vi "SVA 4MV6 P001 CCE histograma colores.vi"(11 "Image":T1) -> (1 "HGB":u8[](array[numeric]), 2 "HGG":u8[](array[numeric]), 3 "HGR":u8[](array[numeric]))   [LabVIEW 2020]
uses:
  <vilib>/vision/Image Controls.llb/IMAQ Image.ctl
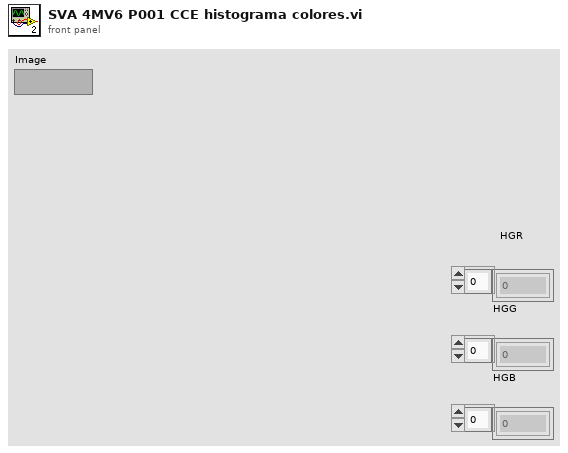
[diagram p1: front panel]
types:
  T1 = typedef "IMAQ Image.ctl" = refnum<image>
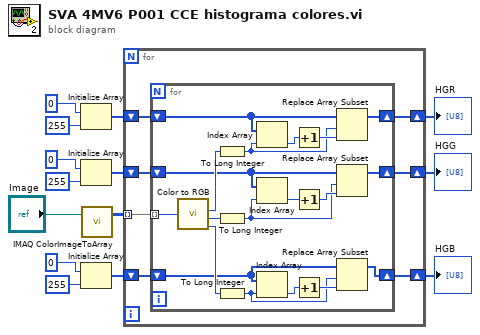
[diagram p0: block diagram]
diagram:
  n1 = Initialize Array(u8 0 ("element"), 255 ("dimension size")) -> (w12:u8[])
  n2 = Initialize Array(u8 0 ("element"), 255 ("dimension size")) -> (w6:u8[])
  n3 = Initialize Array(u8 0 ("element"), 255 ("dimension size")) -> (w5:u8[])
  n4 = call "IMAQ ColorImageToArray"("Image"="Image") -> ("Image Pixels (U32)"=w11:u32[][])  [unwired: 3 in, 2 out]
  n5 = for {
    shift-right: [w20] -> w4
    shift-left: w12 -> [w21]
    tunnel: w11 -> [w19] mode=indexing
    shift-right: [w17] -> w3
    shift-left: w6 -> [w18]
    shift-right: [w15] -> w2
    shift-left: w5 -> [w16]
    n6 = for {
      shift-right: [w37] -> w20
      shift-left: w21 -> [w38]
      tunnel: w19 -> [w36] mode=indexing
      shift-right: [w28] -> w17
      shift-left: w18 -> [w30]
      shift-right: [w22] -> w15
      shift-left: w16 -> [w23]
      n7 = call <vilib>:"Color to RGB.vi"("Color"=w36) -> ("R"=w35:u8, "G"=w29:u8, "B"=w24:u8)  [unwired: 1 out]
      n8 = To Long Integer(number=w35) -> (32bit integer=w34:i32)
      n9 = To Long Integer(number=w29) -> (32bit integer=w31:i32)
      n10 = To Long Integer(number=w24) -> (32bit integer=w25:i32)
      n11 = Index Array(array=w38, index=w34) -> (element=w40:u8)
      n12 = Index Array(array=w30, index=w31) -> (element=w33:u8)
      n13 = Index Array(array=w23, index=w25) -> (element=w27:u8)
      n14 = Increment(x=w40) -> (x+1=w39:u8)
      n15 = Increment(x=w33) -> (x+1=w32:u8)
      n16 = Increment(x=w27) -> (x+1=w26:u8)
      n17 = Replace Array Subset(array=w38, new element=w39, index=w34) -> (w37:u8[])
      n18 = Replace Array Subset(array=w30, new element=w32, index=w31) -> (w28:u8[])
      n19 = Replace Array Subset(array=w23, new element=w26, index=w25) -> (w22:u8[])
    }
  }
  "HGR" <- w4
  "HGG" <- w3
  "HGB" <- w2
